vi "Validate Metadata.vi"(8 "error in":errorcluster, 11 "measurement plugin service in":refnum<class "Measurement Plugin Service.lvclass">) -> (0 "error out":errorcluster, 3 "measurement plugin service out":refnum<class "Measurement Plugin Service.lvclass">)   [LabVIEW 2020, in "MeasurementLink Measurement Server.lvlib"]
uses:
  MeasurementLink Measurement Server.lvlib
  Measurement Plugin Service/Measurement Plugin Service.lvclass
  Error Strings Global Internal.vi
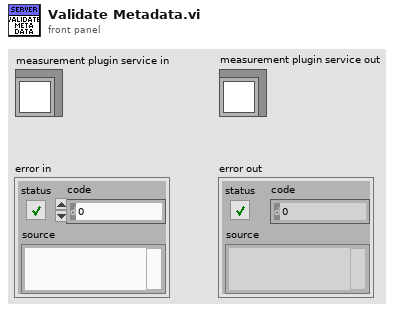
[diagram p1: front panel]
types:
  T1 = typedef "MeasurementLink Measurement Server.lvlib/Measurement Plugin Service.lvclass/Plugin Paths.ctl" = cluster{"get measurement details VI path":path, "get type specializations VI path":path, "get UI details VI path":path, "measurement logic VI path":path, "measurement configuration ctl path":path, "measurement results ctl path":path}
  T2 = typedef "MeasurementLink Measurement Server.lvlib/Parameter Type Specialization.ctl" = cluster{"parameter name":string, "type specialization":T3, "annotations":cluster{"key":T4, "value":string}[]}
  T3 = typedef "MeasurementLink Measurement Server.lvlib/Type Specialization.ctl" = enum16{"none", "pin", "path", "enum"}
  T4 = typedef "MeasurementLink Measurement Server.lvlib/Type Specialization Key.ctl" = enum16{"none", "pin.instrument_type", "enum.values"}
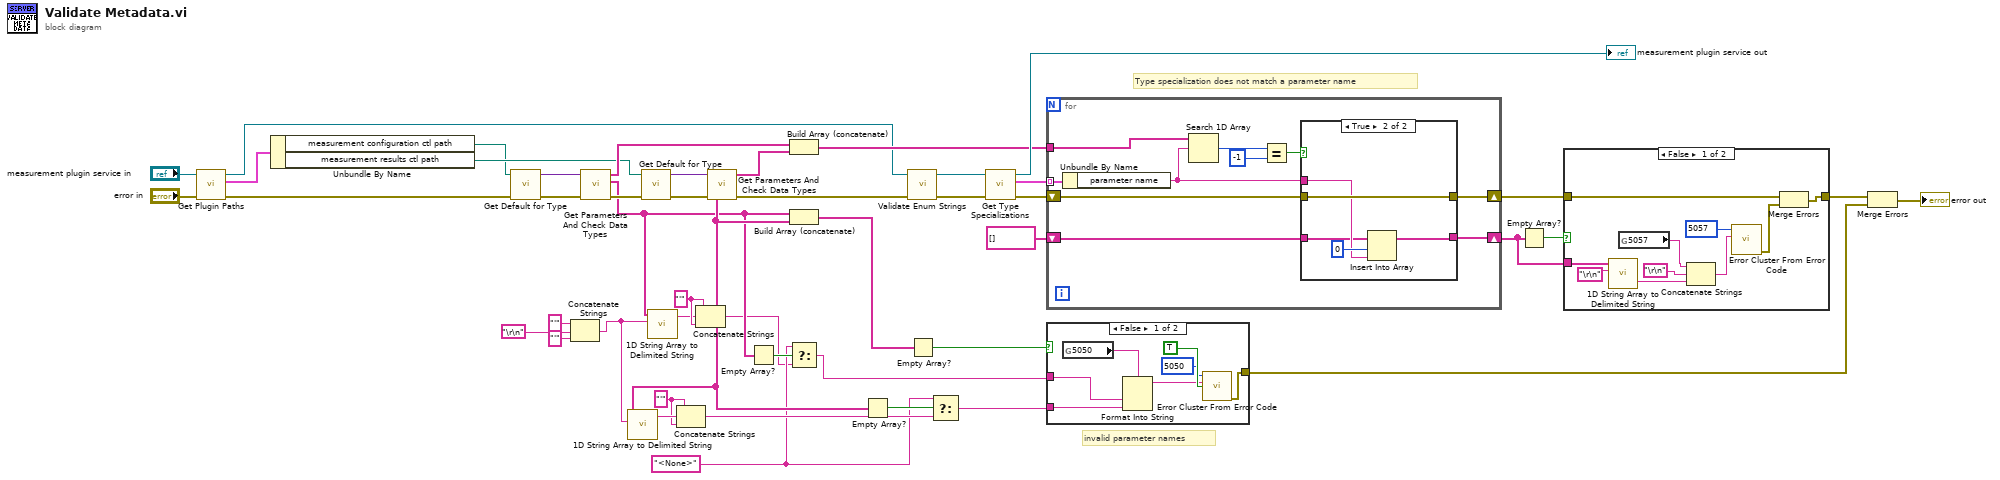
[diagram p0: block diagram]
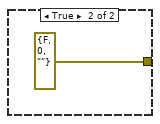
[diagram p2: hidden frame]
diagram:
  w7 = "<None>" ("t")
  w15 = "'" ("string")
  w16 = "'" ("string")
  # "Type specialization does not match a parameter name"
  # "invalid parameter names"
  n1 = call-dynamic "Get Plugin Paths.vi"("error in"="error in", "measurement plugin service in"="measurement plugin service in") -> ("error out"=w25:errorcluster, "plugin paths"=w42:T1, "measurement plugin service out"=w20:refnum<class "Measurement Plugin Service.lvclass">)  [unwired: 7 in]
  n2 = Unbundle By Name(w42) -> ("measurement configuration ctl path"=w28:path, "measurement results ctl path"=w29:path)
  n3 = call "Get Default for Type.vi"("error in"=w25, "path of type"=w28) -> ("error out"=w24:errorcluster, "default for type"=w27:variant)  [unwired: 8 in]
  n4 = Concatenate Strings("'" ("string"), "\r\n", "'" ("string")) -> (w1:string)
  n5 = call "Get Parameters And Check Data Types.vi"("error in"=w24, "variant"=w27) -> ("error out"=w23:errorcluster, "parameters with invalid type"=w9:string[], "parameter names"=w32:string[])  [unwired: 7 in]
  n6 = call "Get Default for Type.vi"("error in"=w23, "path of type"=w29) -> ("error out"=w22:errorcluster, "default for type"=w26:variant)  [unwired: 8 in]
  n7 = call <vilib>:"1D String Array to Delimited String.vi"("delimiter"=w1, "string array"=w9) -> ("delimited string"=w14:string)  [unwired: 9 in]
  n8 = Concatenate Strings(w15, w14, w15) -> (w6:string)
  n9 = call "Get Parameters And Check Data Types.vi"("error in"=w22, "variant"=w26) -> ("error out"=w21:errorcluster, "parameters with invalid type"=w13:string[], "parameter names"=w31:string[])  [unwired: 7 in]
  n10 = call <vilib>:"1D String Array to Delimited String.vi"("delimiter"=w1, "string array"=w13) -> ("delimited string"=w17:string)  [unwired: 9 in]
  n11 = Concatenate Strings(w16, w17, w16) -> (w11:string)
  n12 = Empty Array?(array=w9) -> (empty?=w8:bool)
  n13 = Build Array (concatenate)(w32, w31) -> (w30:string[])
  n14 = Build Array (concatenate)(w9, w13) -> (w33:string[])
  n15 = Select(t=w7, s=w8, f=w6) -> (s? t:f=w5:string)
  n16 = Empty Array?(array=w13) -> (empty?=w12:bool)
  n17 = call "Validate Enum Strings.vi"("error in"=w21, "measurement plugin service in"=w20) -> ("error out"=w18:errorcluster, "measurement plugin service out"=w19:refnum<class "Measurement Plugin Service.lvclass">)  [unwired: 8 in]
  n18 = Empty Array?(array=w33) -> (empty?=w37:bool)
  n19 = Select(t=w7, s=w12, f=w11) -> (s? t:f=w10:string)
  n20 = call-dynamic "Get Type Specializations.vi"("error in"=w18, "measurement plugin service in"=w19) -> ("error out"=w46:errorcluster, "type specializations"=w45:T2[], "measurement plugin service out"=→"measurement plugin service out":refnum<class "Measurement Plugin Service.lvclass">)  [unwired: 7 in]
  n21 = for {
    tunnel: w45 -> [w57] mode=indexing
    shift-right: [w51] -> w38
    shift-left: w46 -> [w52]
    tunnel: w30 -> [w56]
    shift-right: [w48] -> w41
    shift-left: string[] [] -> [w50]
    n22 = Unbundle By Name(w57) -> ("parameter name"=w49:string)
    n23 = Search 1D Array(1D array=w56, element=w49) -> (index of element=w55:i32)  [unwired: 1 in]
    n24 = Equal?(x=w55, y=-1) -> (x = y?=w53:bool)
    n25 = case shown="True" w53 {
      tunnel: w52 -> [w59 w64]
      tunnel: [w59 w64] -> w51
      tunnel: w50 -> [w58 w61]
      tunnel: w49 -> [_ w62]
      tunnel: [w58 w60] -> w48
      frame False {
      }
      frame True {
        n26 = Insert Into Array(array=w61, index=0, new element=w62) -> (w60:string[])
      }
    }
  }
  n27 = case shown="False" w37 {
    tunnel: [w71 errorcluster {"status"=FALSE, "code"=0, "source"=""} ("error out")] -> w34
    tunnel: w5 -> [w68 _]
    tunnel: w10 -> [w65 _]
    frame False {
      n28 = global read "Error Strings Global Internal.vi" "5050"() -> (w66:string)
      n29 = Format Into String(format string=w66, w68, w65) -> (resulting string=w67:string)  [unwired: 2 in, 1 out]
      n30 = call <vilib>:"Error Cluster From Error Code.vi"("show call chain? (False)"=TRUE, "error message (\"\")"=w67, "error code (0)"=5050) -> ("error out"=w71:errorcluster)  [unwired: 6 in]
    }
    frame True {
    }
  }
  n31 = Empty Array?(array=w41) -> (empty?=w40:bool)
  n32 = case shown="False" w40 {
    tunnel: w41 -> [w79 _]
    tunnel: w38 -> [w74 w83]
    tunnel: [w75 w83] -> w35
    frame False {
      n33 = call <vilib>:"1D String Array to Delimited String.vi"("delimiter"="\r\n", "string array"=w79) -> ("delimited string"=w80:string)  [unwired: 9 in]
      n34 = global read "Error Strings Global Internal.vi" "5057"() -> (w78:string)
      n35 = Concatenate Strings(w78, "\r\n", w80) -> (w76:string)
      n36 = call <vilib>:"Error Cluster From Error Code.vi"("error message (\"\")"=w76, "error code (0)"=5057) -> ("error out"=w73:errorcluster)  [unwired: 7 in]
      n37 = Merge Errors(w74, w73) -> (w75:errorcluster)
    }
    frame True {
    }
  }
  n38 = Merge Errors(w35, w34) -> (→"error out":errorcluster)
